vi "选择留样瓶对话框.vi"() -> (2 "布尔":bool=TRUE, 3 "选择留样瓶":dbl)   [LabVIEW 2016, in "德润超标留样.lvlib"]
uses:
  <vilib>/Utility/miscctls.llb/LVPointTypeDef.ctl
panel:
  in  "取消":bool
  in  "确定":bool
  # "请选择留样瓶号1~12"
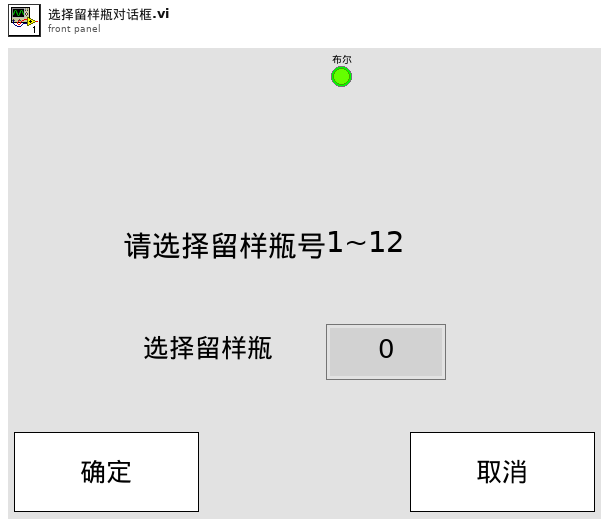
[diagram p1: front panel]
types:
  T1 = typedef "LVPointTypeDef.ctl" = cluster{"Horizontal":i16, "Vertical":i16}
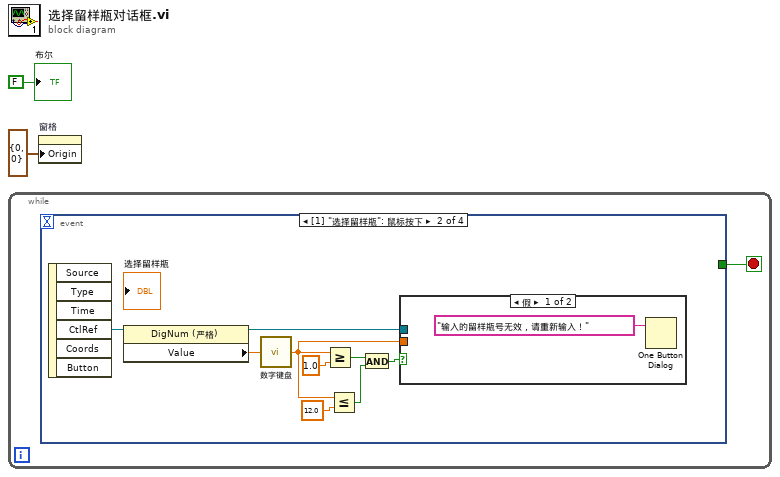
[diagram p0: block diagram]
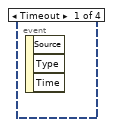
[diagram p2: hidden frame]
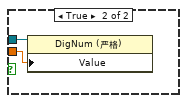
[diagram p3: hidden frame]
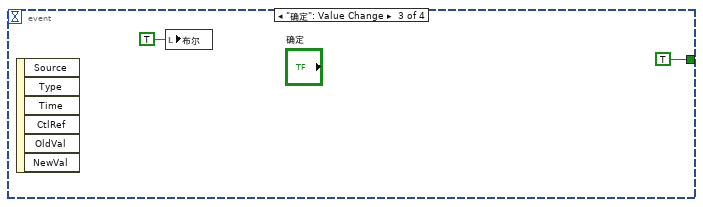
[diagram p4: hidden frame]
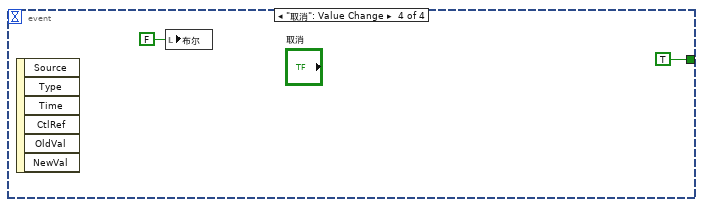
[diagram p5: hidden frame]
diagram:
  n1 = while {
    stop <- w3 stop-if-true
    n2 = event shown="[1] \"选择留样瓶\": 鼠标按下" {
      selector: _ -> [_ _ _ _]
      dyn-events: _ -> [_ _ _ _]
      timeout: _ -> [_ _ _ _]
      tunnel: [_ _ TRUE TRUE] -> w3
      event Timeout {
        n3 = event-data() -> ()  [unwired: 1 in, 3 out]
      }
      event "选择留样瓶": Mouse Down {
        n4 = event-data() -> ("CtlRef"=w12:refnum<vi>)  [unwired: 1 in, 5 out]
        n5 = property class="DigNum (严格)"(reference=w12) -> (reference out=w11:refnum<vi>, "Value"=w10:dbl)  [unwired: 1 in, 1 out]
        n6 = call "数字键盘.vi"("OldNumber"=w10) -> ("NewNumber"=w8:sgl)
        n7 = Greater Or Equal?(x=w8, y=sgl 1.0) -> (x >= y?=w6:bool)
        n8 = Less Or Equal?(x=w8, y=sgl 12.0) -> (x <= y?=w5:bool)
        n9 = And(x=w6, y=w5) -> (x .and. y?=w4:bool)
        n10 = case shown="假" w4 {
          tunnel: w11 -> [_ w15]
          tunnel: w8 -> [_ w14]
          frame False {
            n11 = One Button Dialog(message="输入的留样瓶号无效，请重新输入！" ("消息")) -> ()  [unwired: 1 in, 1 out]
          }
          frame True {
            n12 = property class="DigNum (严格)"(reference=w15, "Value"=w14) -> ()  [unwired: 1 in, 2 out]
          }
        }
      }
      event "确定": Value Change {
        n13 = event-data() -> ()  [unwired: 1 in, 6 out]
        n14 = local write "布尔"(TRUE ("布尔")) -> ()
      }
      event "取消": Value Change {
        n15 = event-data() -> ()  [unwired: 1 in, 6 out]
        n16 = local write "布尔"(FALSE ("布尔")) -> ()
      }
    }
  }
  n17 = property on="窗格" class="Pane"("Origin"=T1 {"Horizontal"=0, "Vertical"=0} ("原点")) -> ()  [unwired: 2 in, 2 out]
  "布尔" <- FALSE ("布尔")
